vi "sous-VI Conversion Nombre Romain en Nombre Arabe.vi"(1 "Enter a ROMAN nomber?":string, 2 "RESULT":bool) -> (0 "Arabic number:":dbl)   [LabVIEW 2019]
panel:
  # "Sous-VI CONVERSION NOMBRE romain EN NOMBRE arabe:"
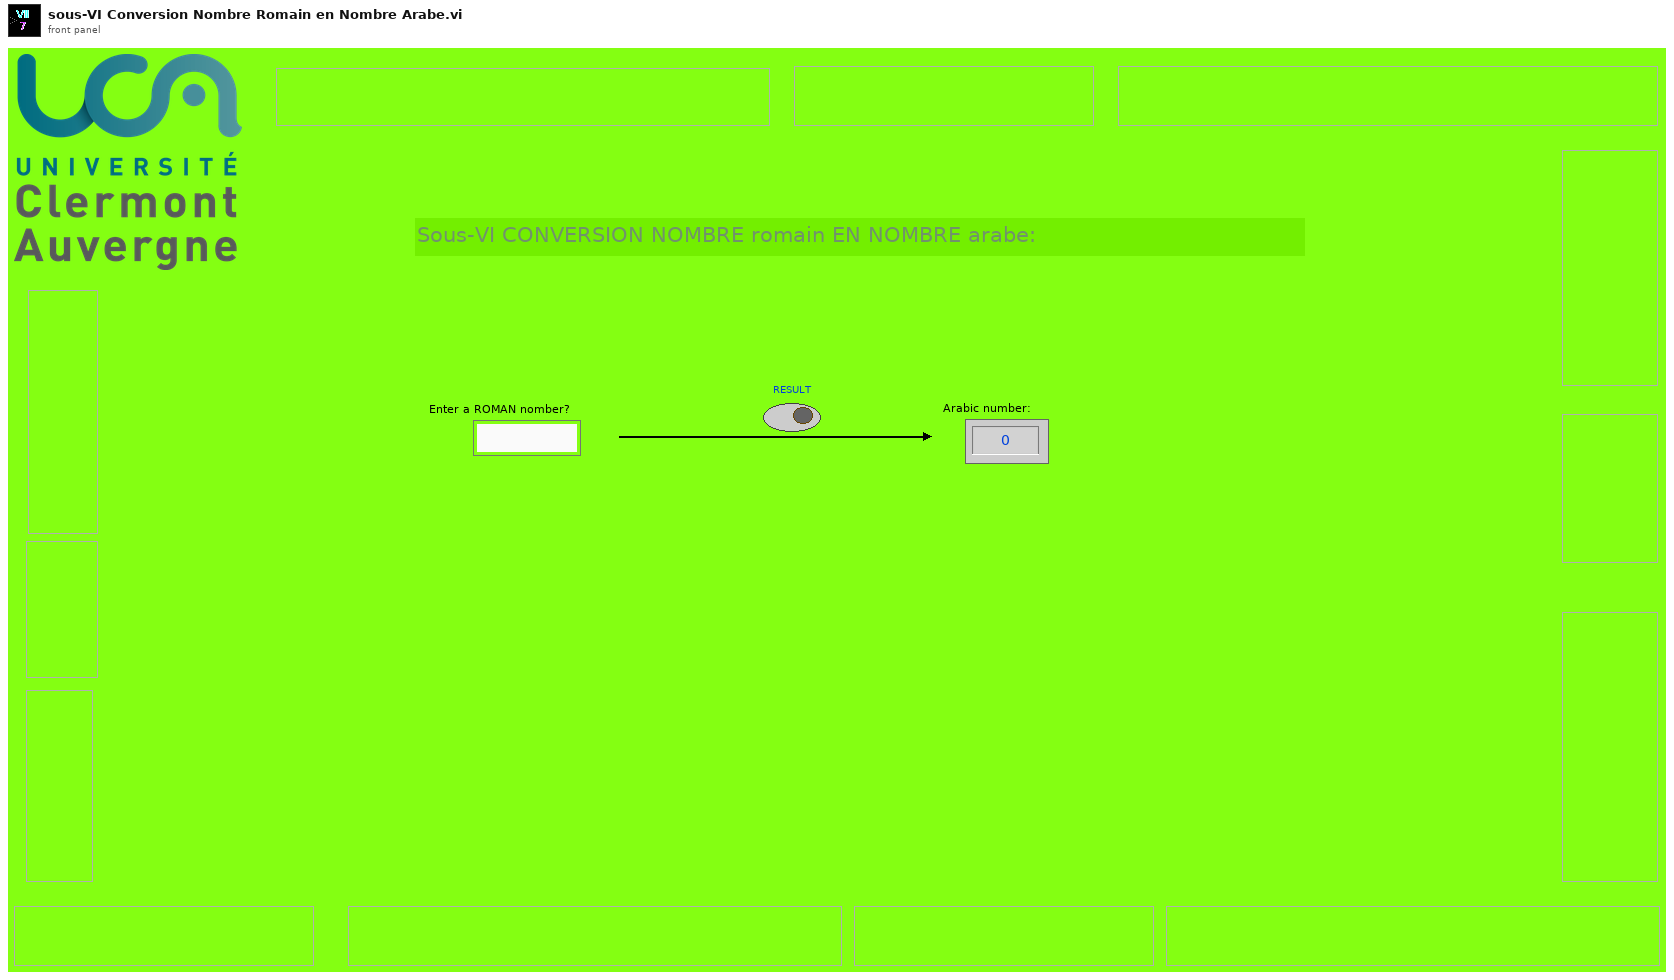
[diagram p1: front panel]
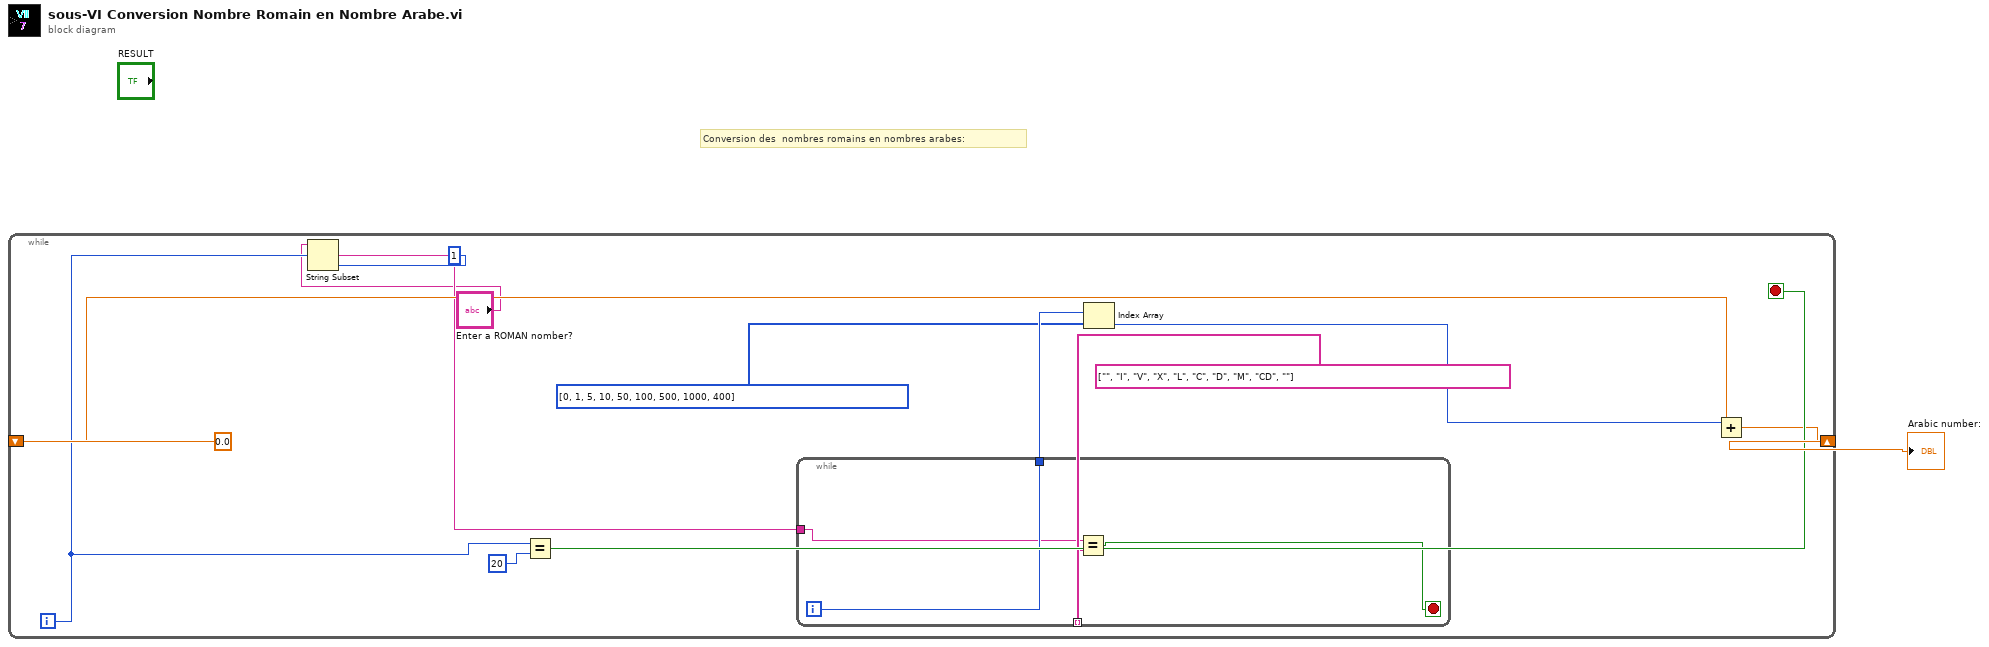
[diagram p0: block diagram]
diagram:
  # "Conversion des  nombres romains en nombres arabes:"
  n1 = while {
    shift-right: [w9] -> w2
    shift-left: 0.0 -> [w14]
    i -> [w10]
    stop <- w12 stop-if-true
    n2 = String Subset(string="Enter a ROMAN nomber?", offset (0)=w10, length (rest)=1 ("length (len. of substring)")) -> (substring=w4:string)
    n3 = Equal?(x=w10, y=20) -> (x = y?=w12:bool)
    n4 = while {
      tunnel: [w18] -> w8
      tunnel: string[] ["", "I", "V", "X", "L", "C", "D", "M", "CD", ""] -> [w17] mode=indexing
      tunnel: w4 -> [w15]
      i -> [w18]
      stop <- w16 stop-if-true
      n5 = Equal?(x=w15, y=w17) -> (x = y?=w16:bool)
    }
    n6 = Index Array(array=i32[] [0, 1, 5, 10, 50, 100, 500, 1000, 400], index=w8) -> (element=w5:i32)
    n7 = Add(x=w5, y=w14) -> (x+y=w9:dbl)
  }
  "Arabic number:" <- w2
